vi "Additive_chi2_kernel.vi"(8 "error in":errorcluster caption="entrée d'erreur", 10 "Y":string[][](array[string]), 11 "X":string[][](array[string])) -> (0 "error out":errorcluster caption="sortie d'erreur", 3 "Data":T1)   [LabVIEW 2020]
doc: "Computes the additive chi-squared kernel between observations in X and Y\n\nThe chi-squared kernel is computed between each pair of rows in X and Y. X and Y have to be non-negative. This kernel is most commonly applied to histograms.\n\nThe chi-squared kernel is given by :\n\nk(x, y) = -Sum [(x - y)^2 / (x + y)]\n\nIt can be interpreted as a weighted difference per entry.\n\nParameters : \n\n- X : array-like of shape (n_samples_X, n_features)\nYarray of shape (n_samples_Y, n_features)\n\nReturns : \n\n- kernel_matrix : array of shape (n_samples_X, n_samples_Y)"
uses:
  Additive_chi2_kernel.lvclass
panel:
  out "Additive_chi2_kernel.lvclass":refnum<class "Additive_chi2_kernel.lvclass">
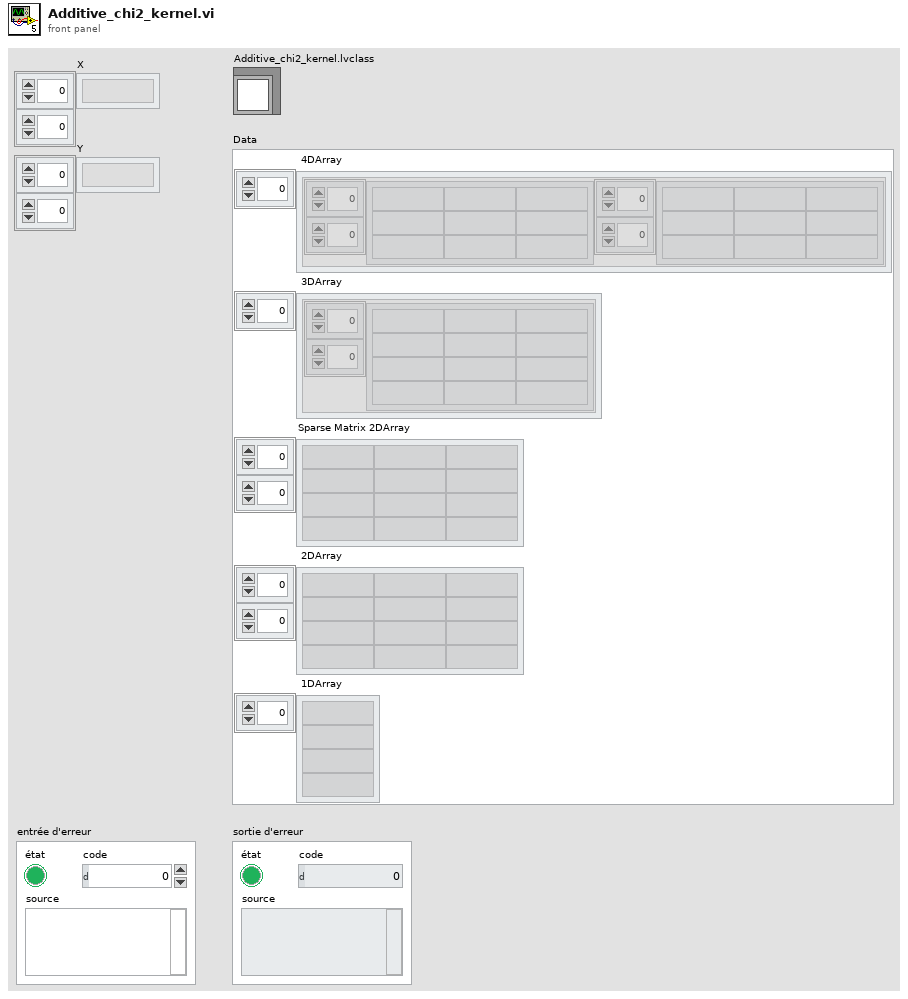
[diagram p1: front panel]
types:
  T1 = cluster{" 4DArray":cluster{"1":string[][], "2":string[][]}[], " 3DArray":cluster{"Tableau":string[][]}[], "Sparse Matrix 2DArray":string[][], " 2DArray":string[][], " 1DArray":string[]}
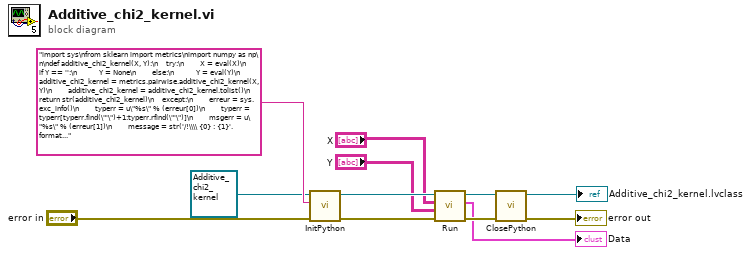
[diagram p0: block diagram]
diagram:
  n1 = call-dynamic "InitPython.vi"("error in (no error)"="error in", "Python Instruction"="import sys\nfrom sklearn import metrics\nimport numpy as np\n\ndef additive_chi2_kernel(X, Y):\n    try:\n        X = eval(X)\n        if Y == '':\n           Y = None\n        else:\n           Y = eval(Y)\n        additive_chi2_kernel = metrics.pairwise.additive_chi2_kernel(X, Y)\n        additive_chi2_kernel = additive_chi2_kernel.tolist()\n        return str(additive_chi2_kernel)\n    except:\n        erreur = sys.exc_info()\n        typerr = u\"%s\" % (erreur[0])\n        typerr = typerr[typerr.find(\"'\")+1:typerr.rfind(\"'\")]\n        msgerr = u\"%s\" % (erreur[1])\n        message = str('/!\\\\ {0} : {1}'. format(typerr,msgerr))\n        return message", "Scikit-learn en entrée"=refnum<class "Additive_chi2_kernel.lvclass"> refnum ("Additive_chi2_kernel.lvclass")) -> ("error out"=w8:errorcluster, "Scikit-learn en sortie"=w9:refnum<class "Additive_chi2_kernel.lvclass">)  [unwired: 7 in]
  n2 = call-dynamic "Run.vi"("error in (no error)"=w8, "Y"="Y", "X"="X", "Additive_chi2_kernel.lvclass"=w9) -> ("error out"=w6:errorcluster, "Data"=→"Data":T1, "Additive_chi2_kernel.lvclass"=w7:refnum<class "Additive_chi2_kernel.lvclass">)  [unwired: 5 in]
  n3 = call-dynamic "ClosePython.vi"("error in (no error)"=w6, "Scikit-learn en entrée"=w7) -> ("error out"=→"error out":errorcluster, "Scikit-learn en sortie"=→"Additive_chi2_kernel.lvclass":refnum<class "Additive_chi2_kernel.lvclass">)  [unwired: 8 in]
